vi "Alias2Child.vi"(8 "error in":errorcluster, 10 "Alias":string) -> (0 "error out":errorcluster, 3 "Instrument out":refnum<class "Instrument.lvclass">)   [LabVIEW 2014, in "Instrument.lvclass"]
uses:
  Instrument.lvclass
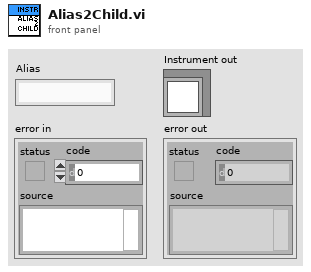
[diagram p1: front panel]
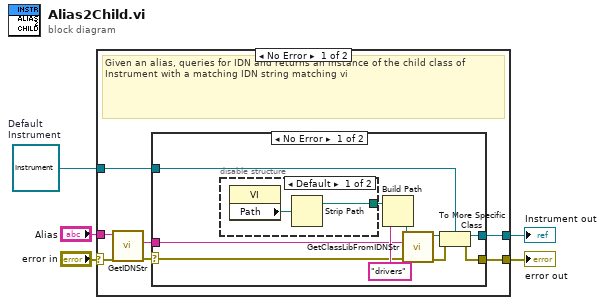
[diagram p0: block diagram]
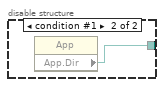
[diagram p2: hidden frame]
diagram:
  w3 = refnum<class "Instrument.lvclass"> refnum  # Default Instrument
  n1 = case shown="No Error" "error in" {
    selector: "error in" -> [w6 w29]
    tunnel: "Alias" -> [w7 _]
    tunnel: [w11 w28] -> w2
    tunnel: [w12 w29] -> w1
    tunnel: w3 -> [w8 w28]
    frame No Error {
      # "Given an alias, queries for IDN and returns an instance of the child class of Instrument with a matching IDN string matching vi"
      n2 = call "GetIDNStr.vi"("error in"=w6, "Alias"=w7) -> ("error out"=w10:errorcluster, "Model ID String"=w9:string)  [unwired: 8 in]
      n3 = case shown="No Error" w10 {
        selector: w10 -> [w19 w27]
        tunnel: [w16 w27] -> w12
        tunnel: [w14 w26] -> w11
        tunnel: w9 -> [w20 _]
        tunnel: w8 -> [w15 w26]
        frame No Error {
          n4 = disable-structure shown="Default" {
            disable-tunnel: [w23 w25] -> w13
            frame condition #0 (active) {
              n5 = property class="VI"() -> ("Path"=w24:path)  [unwired: 2 in, 2 out]
              n6 = Strip Path(path=w24) -> (stripped path=w23:path)  [unwired: 1 out]
            }
            frame condition #1 {
              n7 = property class="App"() -> ("App.Dir"=w25:path)  [unwired: 2 in, 2 out]
            }
          }
          n8 = Build Path(base path=w13, name or relative path="drivers") -> (appended path=w21:path)
          n9 = call "GetClassLibFromIDNStr.vi"("error in"=w19, "IDNStr"=w20, "Driver folder"=w21) -> ("error out"=w17:errorcluster, "object"=w18:refnum<class>)  [unwired: 7 in]
          n10 = To More Specific Class(target class=w15, reference=w18, error in=w17) -> (specific class reference=w14:refnum<class "Instrument.lvclass">, error out=w16:errorcluster)
        }
        frame Error {
        }
      }
    }
    frame Error {
    }
  }
  "error out" <- w1
  "Instrument out" <- w2
